vi "Size (ARGB).vi"(8 "error in (no error)":errorcluster, 11 "ARGB Image in":T1) -> (0 "error out":errorcluster, 2 "Image Size":T2, 3 "ARGB Image":T1)   [LabVIEW 2020, in "image.lvlib"]
doc: "Get the Size of the Image."
uses:
  image.lvlib
  ARGB Image.ctl
  common/Image Size (Integer).ctl
  69a1505b-b287-44ed-9ef9-f10ed7b260f4.vi
  common/common.lvlib
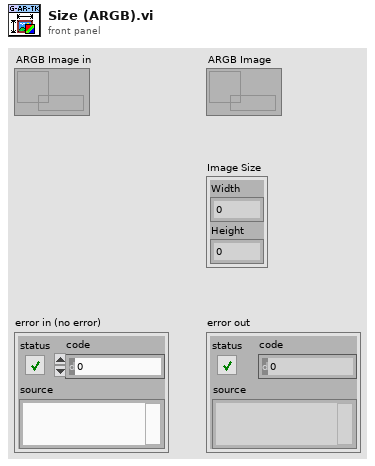
[diagram p1: front panel]
types:
  T1 = typedef "image.lvlib/ARGB Image.ctl" = refnum<data-value>
  T2 = typedef "common.lvlib/Image Size (Integer).ctl" = cluster{"Width":u16, "Height":u16}
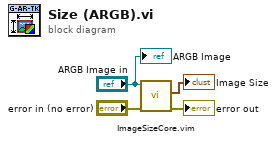
[diagram p0: block diagram]
diagram:
  n1 = call "ImageSizeCore.vim"("error in (no error)"="error in (no error)", "Image"="ARGB Image in") -> ("error out"=→"error out":errorcluster, "Image Size"=→"Image Size":T2)  [unwired: 8 in]
  "ARGB Image" <- "ARGB Image in"
